vi "FindErrorsUsingText.vi"(8 "ErrorIn":errorcluster caption="Error In(no Error)", 9 "SearchTexts":string[](array[string]), 11 "ReferenceIn":refnum<class "ErrorDefinitionSQLite.lvclass"> caption="Reference In") -> (0 "ErrorOut":errorcluster caption="Error Out", 1 "Errors":T1, 3 "ReferenceOut":refnum<class "ErrorDefinitionSQLite.lvclass"> caption="Reference Out")   [LabVIEW 2018, in "ErrorDefinitionSQLite.lvclass"]
uses:
  <userlib>/_express/CustomErrorCreator/ErrorDefinitionSQLite/ErrorDefinitionSQLite.lvclass
  <userlib>/_express/CustomErrorCreator/ErrorDefinitionSQLite/ErrorContent.ctl
  <vilib>/drjdpowell/SQLite Library/SQL Connection/Open (path).vi
  <vilib>/drjdpowell/SQLite Library/SQL Connection/Open (string).vi
  <vilib>/AdvancedString/Path To Command Line String.vi
  <vilib>/drjdpowell/SQLite Library/SQL Connection/Execute SQL.vi
  <vilib>/drjdpowell/SQLite Library/SQL Connection/Connection.lvclass
  <vilib>/drjdpowell/SQLite Library/SQLite.lvlib
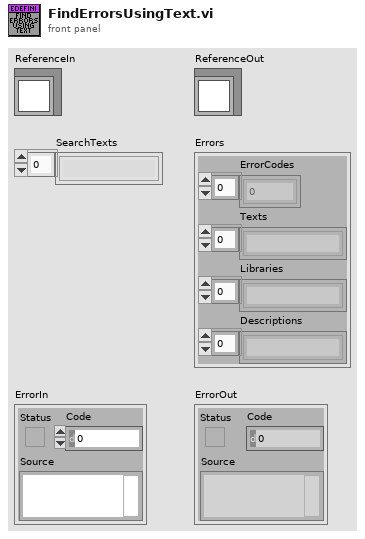
[diagram p1: front panel]
types:
  T1 = typedef "ErrorDefinitionSQLite.lvclass/ErrorContent.ctl" = cluster{"ErrorCodes":i32[], "Texts":string[], "Libraries":string[], "Descriptions":string[]}
  T2 = enum16{"New or existing", "Existing", "Read only"}
  T3 = typedef "ErrorDefinitionSQLite.lvclass/ObjectAttributes.ctl" = cluster{"Path":path}
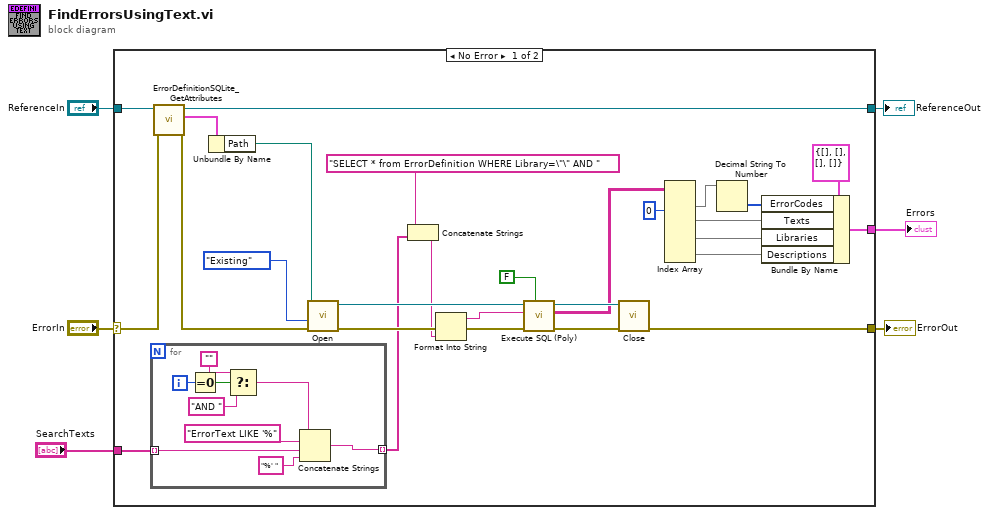
[diagram p0: block diagram]
diagram:
  n1 = case shown="No Error" "ErrorIn" {
    selector: "ErrorIn" -> [w34 w45]
    tunnel: [w20 w45] -> w5
    tunnel: [w32 w44] -> w3
    tunnel: "ReferenceIn" -> [w33 w44]
    tunnel: "SearchTexts" -> [w10 _]
    tunnel: [w11 _] -> w2
    frame No Error {
      n2 = for {
        tunnel: w10 -> [w43] mode=indexing
        tunnel: [w40] -> w8 mode=indexing
        i -> [w39]
        n3 = Equal To 0?(x=w39) -> (x = 0?=w38:bool)
        n4 = Select(t="", s=w38, f="AND " ("string")) -> (s? t:f=w35:string)
        n5 = Concatenate Strings(w35, "ErrorText LIKE '%" ("string"), w43, "%' " ("string")) -> (w40:string)
      }
      n6 = call <userlib>:"ErrorDefinitionSQLite_GetAttributes.vi"("ErrorIn"=w34, "Reference in"=w33) -> ("ErrorOut"=w28:errorcluster, "Data"=w30:T3, "Reference out"=w32:refnum<class "ErrorDefinitionSQLite.lvclass">)  [unwired: 6 in, 1 out]
      n7 = Unbundle By Name(w30) -> ("Path"=w29:path)
      n8 = call-poly <vilib>:"Open.vi"("error in (no error)"=w28, "File Option"=T2."Existing", "db file"=w29) -> ("error out"=w24:errorcluster, "SQLite Connection"=w26:refnum<class "Connection.lvclass">)  [unwired: 7 in]
      n9 = Concatenate Strings("SELECT * from ErrorDefinition WHERE Library=\"\" AND " ("SQL"), w8) -> (w7:string)
      n10 = Format Into String(error in=w24, w7) -> (resulting string=w25:string, error out=w23:errorcluster)  [unwired: 2 in]
      n11 = call-poly <vilib>:"Execute SQL (Poly).vi"("Use SAVEPOINT"=FALSE, "error in (no error)"=w23, "SQL"=w25, "SQLite Connection in"=w26) -> ("error out"=w21:errorcluster, "Result Set"=w19:string[][], "SQLite Connection"=w22:refnum<class "Connection.lvclass">)  [unwired: 4 in, 1 out]
      n12 = call-dynamic "Close.vi"("error in (no error)"=w21, "SQLite Connection in"=w22) -> ("error out"=w20:errorcluster)  [unwired: 9 in]
      n13 = Index Array(array=w19, index (col) #1=0 ("disabled index (col)")) -> (element #1=w13:string[], element #2=w14:string[], element #3=w15:string[], element #4=w16:string[])  [unwired: 7 in]
      n14 = Decimal String To Number(string=w13) -> (number=w12:i32[])  [unwired: 2 in, 1 out]
      n15 = Bundle By Name(cluster=T1 {"ErrorCodes"=[], "Texts"=[], "Libraries"=[], "Descriptions"=[]} ("Errors"), "ErrorCodes"=w12, "Texts"=w14, "Libraries"=w15, "Descriptions"=w16) -> (w11:T1)
    }
    frame Error {
    }
  }
  "ErrorOut" <- w5
  "ReferenceOut" <- w3
  "Errors" <- w2
